vi "FourCC Int to String.vi"(10 "error in (no error)":errorcluster, 11 "fourCC Int":i32=1196444237) -> (2 "error out":errorcluster, 3 "fourCC String":string)   [LabVIEW 2014]
doc: "Help VI to convert the FourCC String to Int and back"
uses:
  Dependencies/x86/MSC I Process32.dll
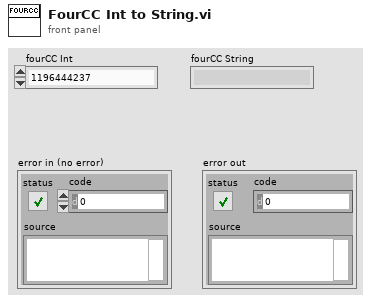
[diagram p1: front panel]
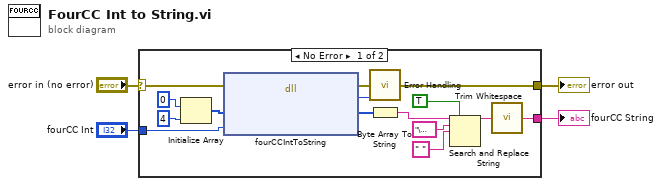
[diagram p0: block diagram]
diagram:
  n1 = case shown="No Error" "error in (no error)" {
    selector: "error in (no error)" -> [w17 w20]
    tunnel: [w16 w20] -> w4
    tunnel: [w6 _] -> w2
    tunnel: "fourCC Int" -> [w5 _]
    frame No Error {
      n2 = Initialize Array(u8 0, 4 ("dimension size")) -> (w12:u8[])
      n3 = dll-call lib="C:/Users/MSC/LabVIEW Projekte/LV 2014/MSC I-Process/user.lib/MSC-I Process/Dependencies/x86/MSC I Process*.dll" fn="fourCCIntToString"(error in=w17, "fourCCString"=w12, "fourCCInt"=w5) -> (error out=w19:errorcluster, "error"=w18:i32, "fourCCString"=w15:u8[])  [unwired: 3 in, 1 out]
      n4 = call "Error Handling.vi"("error in (no error)"=w19, "return type"=w18) -> ("error out"=w16:errorcluster)  [unwired: 12 in, 1 out]
      n5 = Byte Array To String(unsigned byte array=w15) -> (string=w7:string)
      n6 = Search and Replace String(replace all?=TRUE ("replace all? (F)"), input string=w7, search string="\u0000", replace string=" " ("replace string (\"\")")) -> (result string=w8:string)  [unwired: 4 in, 3 out]
      n7 = call <vilib>:"Trim Whitespace.vi"("string"=w8) -> ("trimmed string"=w6:string)  [unwired: 1 in]
    }
    frame Error {
    }
  }
  "error out" <- w4
  "fourCC String" <- w2
